vi "Untitled 4.vi"(11 "reference":refnum<vi>) -> ()   [LabVIEW 2018, in "Image Process.lvclass"]
uses:
  Image Process.lvclass
panel:
  in  "Value":variant
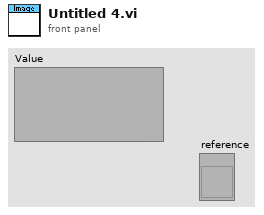
[diagram p1: front panel]
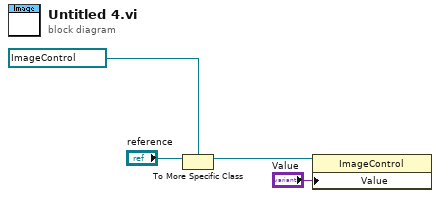
[diagram p0: block diagram]
diagram:
  n1 = To More Specific Class(target class=refnum<vi> refnum ("reference"), reference="reference") -> (specific class reference=w2:refnum<vi>)  [unwired: 1 in, 1 out]
  n2 = property class="ImageControl"(reference=w2, "Value"="Value") -> ()  [unwired: 1 in, 2 out]
